vi "Pid.vi"(0 "Boolean":bool, 7 "Right Motor Power":dbl, 9 "Left Motor Power":dbl, 11 "Cluster":T1) -> (8 "Right Motor Output":dbl, 10 "Left Motor Output":dbl)   [LabVIEW 2013]
uses:
  Drive Train Metrics.ctl
  CmdFlag.ctl
  <vilib>/addons/control/pid/pid.llb/PID (DBL).vi
  <vilib>/addons/control/pid/NI_PID_pid.lvlib
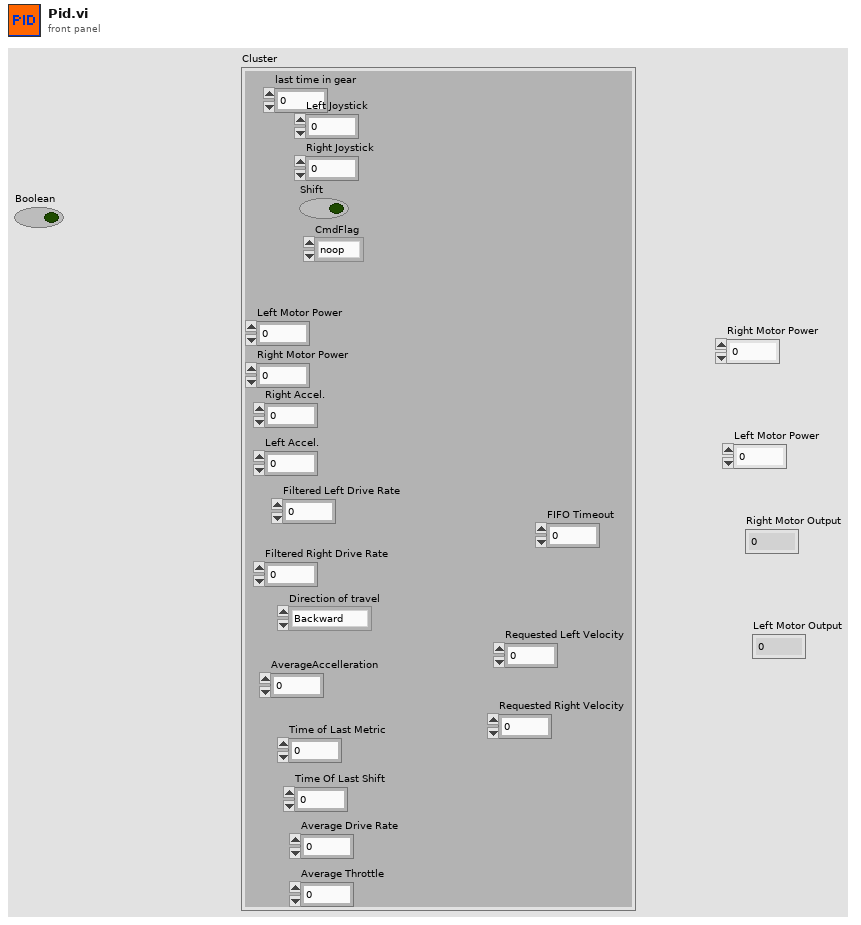
[diagram p1: front panel]
types:
  T1 = typedef "Drive Train Metrics.ctl" = cluster{"last time in gear":u32, "Shift":bool, "Right Joystick":dbl, "Left Joystick":dbl, "CmdFlag":T2, "Right Motor Power":dbl, "Left Motor Power":dbl, "Right Accel.":dbl, "Left Accel.":dbl, "Filtered Left Drive Rate":dbl, "Filtered Right Drive Rate":dbl, "Direction of travel":enum16{"Backward", "Forward", "Spin"}, "AverageAccelleration":dbl, "Time of Last Metric":u32, "Time Of Last Shift":dbl, "Average Drive Rate":dbl, "Average Throttle":dbl, "FIFO Timeout":i32, "Requested Left Velocity":dbl, "Requested Right Velocity":dbl}
  T2 = typedef "CmdFlag.ctl" = enum16{"noop", "suspend", "resume"}
  T3 = cluster{"proportional gain (Kc)":dbl, "integral time (Ti, min)":dbl, "derivative time (Td, min)":dbl}
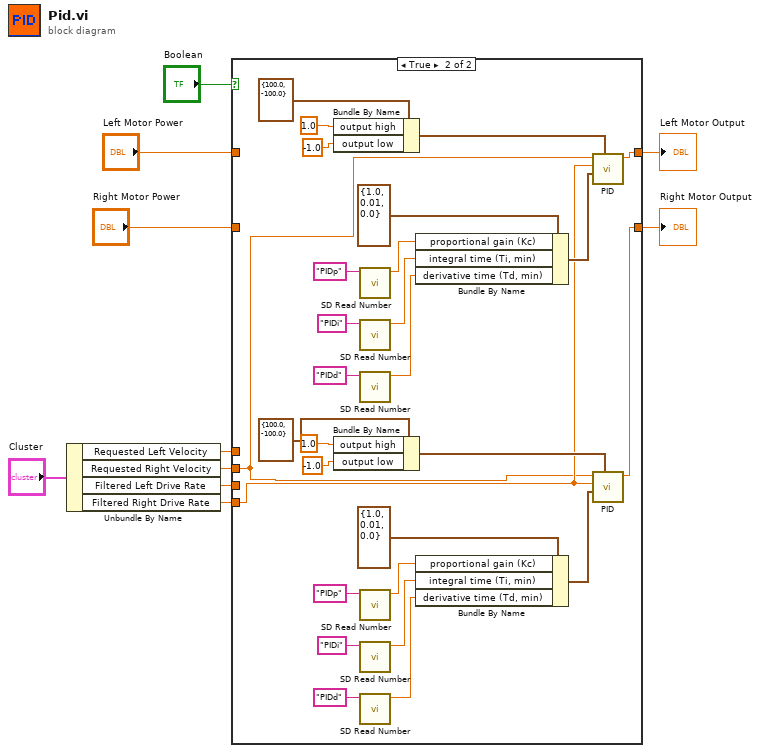
[diagram p0: block diagram]
diagram:
  n1 = Unbundle By Name("Cluster") -> ("Requested Left Velocity"=w1:dbl, "Requested Right Velocity"=w4:dbl, "Filtered Left Drive Rate"=w2:dbl, "Filtered Right Drive Rate"=w3:dbl)
  n2 = case shown="True" "Boolean" {
    tunnel: "Right Motor Power" -> [w12 _]
    tunnel: [w12 w15] -> w7
    tunnel: "Left Motor Power" -> [w11 _]
    tunnel: [w11 w18] -> w6
    tunnel: w4 -> [_ w13]
    tunnel: w3 -> [_ w14]
    tunnel: w2 -> [_ _]
    tunnel: w1 -> [_ _]
    frame False {
    }
    frame True {
      n3 = Bundle By Name(cluster=cluster{"output high":dbl, "output low":dbl} {"output high"=100.0, "output low"=-100.0} ("output range"), "output high"=1.0, "output low"=-1.0) -> (w27:cluster{"output high":dbl, "output low":dbl})
      n4 = Bundle By Name(cluster=cluster{"output high":dbl, "output low":dbl} {"output high"=100.0, "output low"=-100.0} ("output range"), "output high"=1.0, "output low"=-1.0) -> (w17:cluster{"output high":dbl, "output low":dbl})
      n5 = call <vilib>:"SD Read Number.vi"("Name"="PIDp") -> ("Numeric"=w24:dbl)  [unwired: 8 in, 2 out]
      n6 = call <vilib>:"SD Read Number.vi"("Name"="PIDi") -> ("Numeric"=w23:dbl)  [unwired: 8 in, 2 out]
      n7 = call <vilib>:"SD Read Number.vi"("Name"="PIDd") -> ("Numeric"=w22:dbl)  [unwired: 8 in, 2 out]
      n8 = call <vilib>:"SD Read Number.vi"("Name"="PIDp") -> ("Numeric"=w36:dbl)  [unwired: 8 in, 2 out]
      n9 = call <vilib>:"SD Read Number.vi"("Name"="PIDi") -> ("Numeric"=w35:dbl)  [unwired: 8 in, 2 out]
      n10 = call <vilib>:"SD Read Number.vi"("Name"="PIDd") -> ("Numeric"=w34:dbl)  [unwired: 8 in, 2 out]
      n11 = Bundle By Name(cluster=T3 {"proportional gain (Kc)"=1.0, "integral time (Ti, min)"=0.01, "derivative time (Td, min)"=0.0} ("PID gains"), "proportional gain (Kc)"=w24, "integral time (Ti, min)"=w23, "derivative time (Td, min)"=w22) -> (w25:T3)
      n12 = Bundle By Name(cluster=T3 {"proportional gain (Kc)"=1.0, "integral time (Ti, min)"=0.01, "derivative time (Td, min)"=0.0} ("PID gains"), "proportional gain (Kc)"=w36, "integral time (Ti, min)"=w35, "derivative time (Td, min)"=w34) -> (w16:T3)
      n13 = call-poly <vilib>:"PID.vi"("output range"=w27, "PID gains"=w25, "process variable"=w14, "setpoint"=w13) -> ("output"=w18:dbl)  [unwired: 6 in, 1 out]
      n14 = call-poly <vilib>:"PID.vi"("output range"=w17, "PID gains"=w16, "process variable"=w14, "setpoint"=w13) -> ("output"=w15:dbl)  [unwired: 6 in, 1 out]
    }
  }
  "Right Motor Output" <- w7
  "Left Motor Output" <- w6
